vi "Pixel Pass.vi"(11 "Color Box":u32(colorbox)=6618880) -> (3 "Frames":T1[](array[typedef]))   [LabVIEW 2019, in "LED Matrix Host.lvlib"]
uses:
  LED Matrix Host.lvlib
  Public/Controls/Frame.ctl
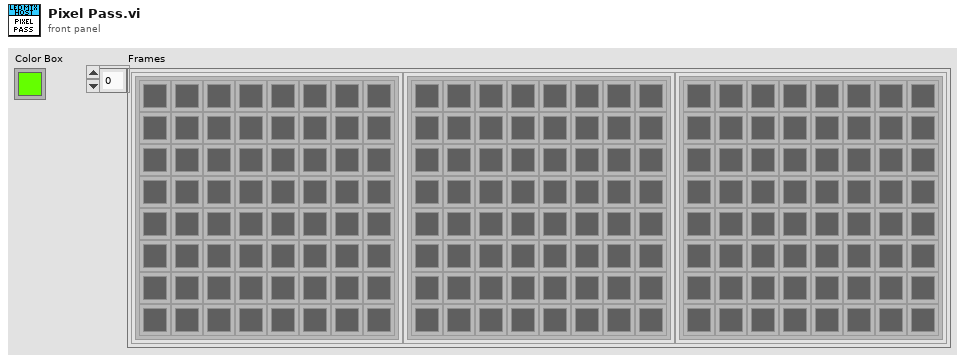
[diagram p1: front panel]
types:
  T1 = typedef "LED Matrix Host.lvlib/Frame.ctl" = cluster{"Matrix":u32[][]}
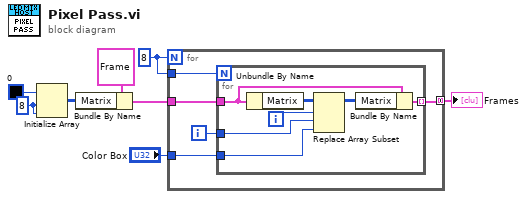
[diagram p0: block diagram]
diagram:
  w2 = 8 ("dimension size")
  w6 = 8
  n1 = Initialize Array(u32 0 ("Color Box"), w2, w2) -> (w3:u32[][])
  n2 = Bundle By Name(cluster=T1 {"Matrix"=[[0, 0, 0, 0, 0, 0, 0, 0], [16777222, 16777222, 0, 0, 0, 0, 0, 0], [0, 0, 0, 0, 0, 0, 0, 0], [0, 0, 0, 0, 0, 0, 0, 0], [0, 0, 0, 0, 0, 0, 0, 0], [0, 0, 0, 0, 0, 0, 0, 0], [0, 0, 0, 0, 0, 0, 0, 0], [16777222, 0, 0, 0, 0, 0, 0, 16777222]]} ("Matrix"), "Matrix"=w3) -> (w1:T1)
  n3 = for {
    N: w6 -> [_]
    tunnel: w1 -> [w13]
    tunnel: "Color Box" -> [w11]
    tunnel: [w12] -> w7 mode=concatenating
    tunnel: w6 -> [w9]
    i -> [w10]
    n4 = for {
      N: w9 -> [_]
      tunnel: w11 -> [w16]
      tunnel: w10 -> [w15]
      tunnel: w13 -> [w19]
      tunnel: [w17] -> w12 mode=indexing
      i -> [w14]
      n5 = Unbundle By Name(w19) -> ("Matrix"=w20:u32[][])
      n6 = Replace Array Subset(array=w20, new element=w16, index (row)=w14, index (col)=w15) -> (w18:u32[][])
      n7 = Bundle By Name(cluster=w19, "Matrix"=w18) -> (w17:T1)
    }
  }
  "Frames" <- w7
